vi "VI_Hierarchy.vi"(8 "error in":errorcluster, 11 "VI Refnum":refnum<vi>) -> (0 "error out":errorcluster, 3 "VI_Hierarchy":refnum<class "VI_Hierarchy.lvclass">)   [LabVIEW 2014, in "VI_Hierarchy.lvclass"]
uses:
  VI_Hierarchy.lvclass
  <vilib>/Utility/traverseref.llb/TRef TravTarget.ctl
  <vilib>/Utility/traverseref.llb/VI Scripting - Traverse.lvlib
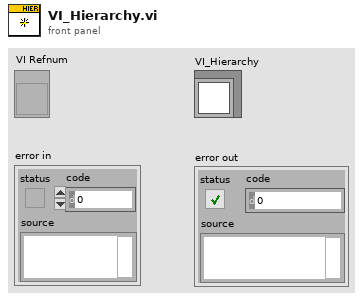
[diagram p1: front panel]
types:
  T1 = typedef "TRef TravTarget.ctl" = enum16{"FP", "BD", "Other"}
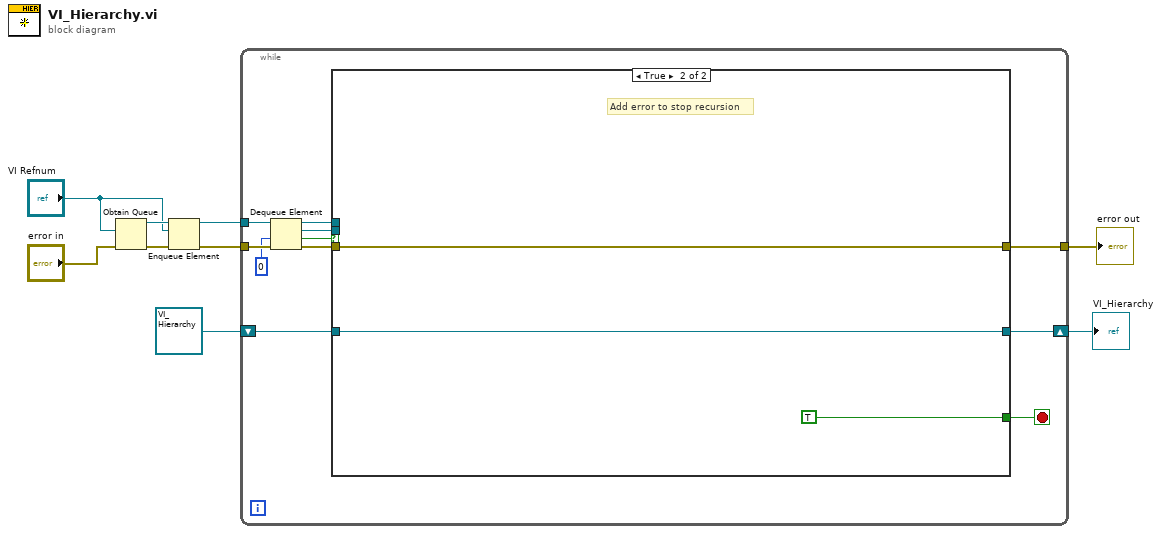
[diagram p0: block diagram]
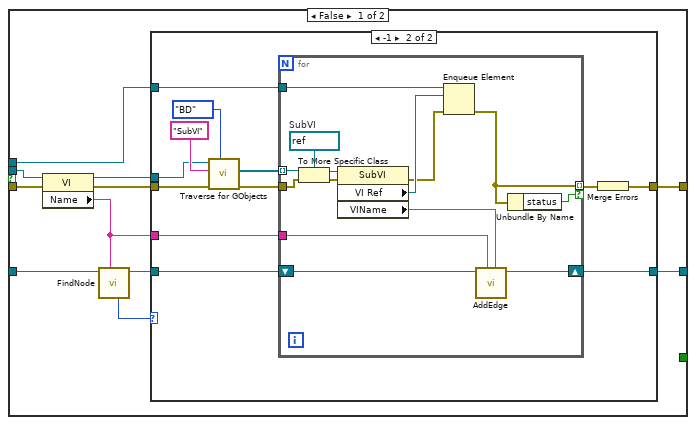
[diagram p2: hidden frame]
diagram:
  n1 = Obtain Queue(element data type="VI Refnum", error in (no error)="error in") -> (queue out=w8:refnum<queue>, error out=w7:errorcluster)  [unwired: 3 in, 1 out]
  n2 = Enqueue Element(queue=w8, element="VI Refnum", error in (no error)=w7) -> (queue out=w6:refnum<queue>, error out=w4:errorcluster)  [unwired: 1 in, 1 out]
  n3 = while {
    tunnel: w6 -> [w20]
    shift-right: [w12] -> w2
    shift-left: refnum<class "VI_Hierarchy.lvclass"> refnum ("VI_Hierarchy") -> [w13]
    tunnel: w4 -> [w15]
    tunnel: [w10] -> w1
    stop <- w11 stop-if-true
    n4 = Dequeue Element(queue=w20, timeout in ms (-1)=0, error in (no error)=w15) -> (queue out=w18:refnum<queue>, element=w17:refnum<vi>, timed out?=w19:bool, error out=w16:errorcluster)
    n5 = case shown="True" w19 {
      tunnel: w18 -> [w27 _]
      tunnel: w17 -> [w30 _]
      tunnel: w16 -> [w31 w60]
      tunnel: w13 -> [w24 w61]
      tunnel: [w26 w61] -> w12
      tunnel: [_ TRUE] -> w11
      tunnel: [w25 w60] -> w10
      frame False {
        n6 = property class="VI"(reference=w30, error in=w31) -> (reference out=w28:refnum<vi>, error out=w29:errorcluster, "Name"=w22:string)
        n7 = call "FindNode.vi"("VI"=w22, "VI_AST in"=w24) -> ("VI_AST out"=w23:refnum<class "VI_Hierarchy.lvclass">, "index"=w21:i32)  [unwired: 6 in]
        n8 = case shown="-1" w21 {
          tunnel: w29 -> [w32 w43]
          tunnel: w28 -> [_ w42]
          tunnel: w27 -> [_ w41]
          tunnel: [w33 w38] -> w26
          tunnel: [w32 w36] -> w25
          tunnel: w23 -> [w33 w35]
          tunnel: w22 -> [_ w34]
          frame Default {
          }
          frame -1 {
            n9 = call <vilib>:"Traverse for GObjects.vi"("Traverse Target"=TRef_TravTarget."BD", "error in (no error)"=w43, "Class Name"="SubVI", "VI Refnum"=w42) -> ("error out"=w39:errorcluster, "References"=w40:refnum<vi>[])  [unwired: 4 in, 2 out]
            n10 = for {
              tunnel: w41 -> [w59]
              tunnel: w40 -> [w58] mode=indexing
              tunnel: w39 -> [w56]
              shift-right: [w49] -> w38
              shift-left: w35 -> [w50]
              tunnel: w34 -> [w51]
              tunnel: [w47] -> w37 mode=indexing if=w46
              w57 = refnum<vi> refnum  # SubVI
              n11 = To More Specific Class(target class=w57, reference=w58, error in=w56) -> (specific class reference=w55:refnum<vi>, error out=w54:errorcluster)
              n12 = property class="SubVI"(reference=w55, error in=w54) -> (error out=w48:errorcluster, "VI Ref"=w53:refnum<vi>, "VIName"=w52:string)  [unwired: 1 out]
              n13 = Enqueue Element(queue=w59, element=w53, error in (no error)=w48) -> (error out=w47:errorcluster)  [unwired: 1 in, 2 out]
              n14 = call "AddEdge.vi"("SubVI"=w52, "VI"=w51, "VI_AST in"=w50) -> ("VI_AST out"=w49:refnum<class "VI_Hierarchy.lvclass">)  [unwired: 6 in]
              n15 = Unbundle By Name(w47) -> ("status"=w46:bool)
            }
            n16 = Merge Errors(w37) -> (w36:errorcluster)
          }
        }
      }
      frame True {
        # "Add error to stop recursion"
      }
    }
  }
  "VI_Hierarchy" <- w2
  "error out" <- w1
